vi "picoquant_process_records.vi"(8 "error in (no error)":errorcluster, 10 "data":u32[](array[numeric]), 11 "picoharp in":refnum<class "picoharp.lvclass">) -> (0 "error out":errorcluster, 2 "data_out":T1, 3 "picoharp out":refnum<class "picoharp.lvclass">)   [LabVIEW 2015, in "picoharp.lvclass"]
uses:
  picoharp.lvclass
  Picoquant_generic/picoquant_data_tdef.ctl
  picoharp.lvclass/picoharp.ctl
  lvoop_dll-master/picoquant_Tmodes.ctl
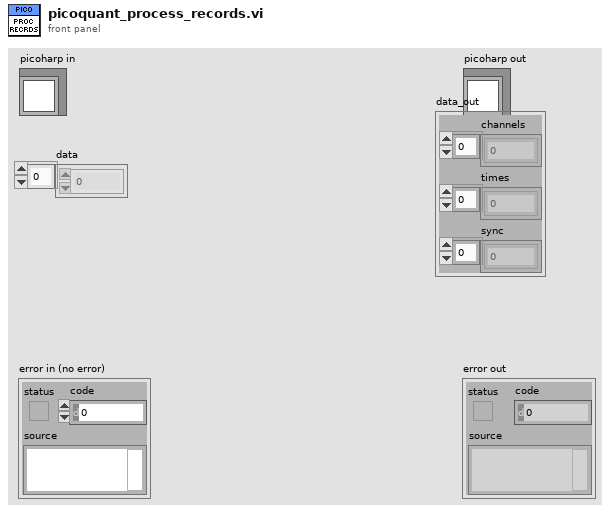
[diagram p1: front panel]
types:
  T1 = typedef "picoquant_data_tdef.ctl" = cluster{"channels":u8[], "times":u64[], "sync":u64[]}
  T2 = typedef "picoquant_Tmodes.ctl" = u16
  T3 = typedef "hpanel_acq_modes.ctl" = u16
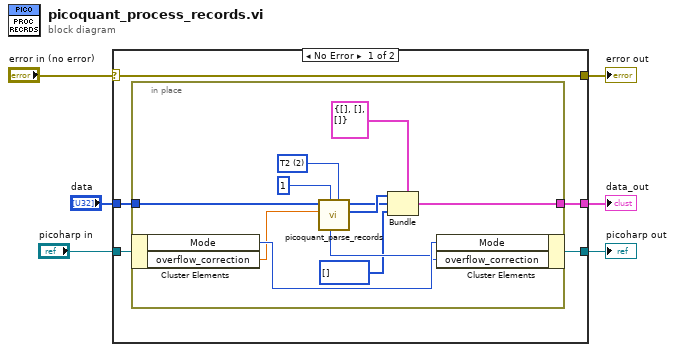
[diagram p0: block diagram]
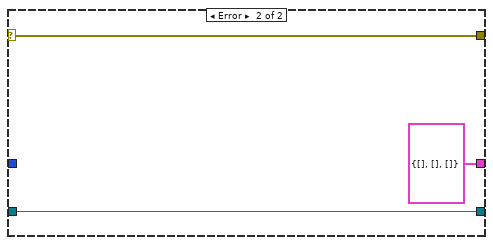
[diagram p2: hidden frame]
diagram:
  n1 = case shown="No Error" "error in (no error)" {
    selector: "error in (no error)" -> [w11 w25]
    tunnel: [w11 w25] -> w3
    tunnel: [w9 w24] -> w2
    tunnel: "picoharp in" -> [w10 w24]
    tunnel: "data" -> [w8 _]
    tunnel: [w7 T1 {"channels"=[], "times"=[], "sync"=[]} ("output cluster")] -> w1
    frame No Error {
      n2 = in-place {
        in-place-border: w8 -> [w18]
        in-place-border: [w13] -> w7
        w12 = T2 2 items=["T2"=2, "T3"=3] ("acq_mode")
        n3 = in-place-cluster #1(w10) -> ("Mode"=w22:T3, "overflow_correction"=w20:dbl)
        n4 = call "picoquant_parse_records.vi"("acq_mode"=w12, "Device"=u8 1 ("device"), "overflow"=w20, "fifo_buffer"=w18) -> ("channels"=w17:u8[], "times"=w16:u64[], "overflow"=w19:u64)  [unwired: 2 in, 3 out]
        n5 = Bundle(cluster=T1 {"channels"=[], "times"=[], "sync"=[]} ("output cluster"), "channels"=w17, "times"=w16, "sync"=u64[] []) -> (w13:T1)
        n6 = in-place-cluster #1("Mode"=w22, "overflow_correction"=w19) -> (w9:refnum<class "picoharp.lvclass">)
      }
    }
    frame Error {
    }
  }
  "error out" <- w3
  "picoharp out" <- w2
  "data_out" <- w1
